vi "Database.GetProductComponentTable.vi"(5 "Idx":i32, 7 "ConnectionString":string, 8 "error in (no error)":errorcluster, 10 "Component_SerialNo":string, 11 "Component_WabcoNo":string) -> (0 "error out":errorcluster, 1 "Prod found":bool, 2 "Product_SerialNo":string, 3 "Product_WabcoNo":string)   [LabVIEW 2016]
uses:
  Tools/Translator/Translator.Message.ctl
  Tools/EventLog/EventLog.EventLevel.ctl
  Tools/EventLog/EventLog.EventSource.ctl
  Tools/EventLog/EventLog.New(array).vi
  <vilib>/addons/database/Connection.llb/DB Tools Open Connec (String).vi
  <vilib>/addons/database/Connection.llb/Conn Execute.vi
  <vilib>/addons/database/Recordset.llb/Rec Fetch Recordset Data (R).vi
  <vilib>/addons/database/Recordset.llb/Rec Destroy - Connection.vi
  Global/ApplicationGlobal.vi
  Tools/EventLog/EventLog.Buffer.vi
  Tools/EventLog/EventLog.File.ReadWrite.vi
  <vilib>/addons/database/NI_Database_API.lvlib
panel:
  in  "Data":i32(listbox)
  out "sql statement":string
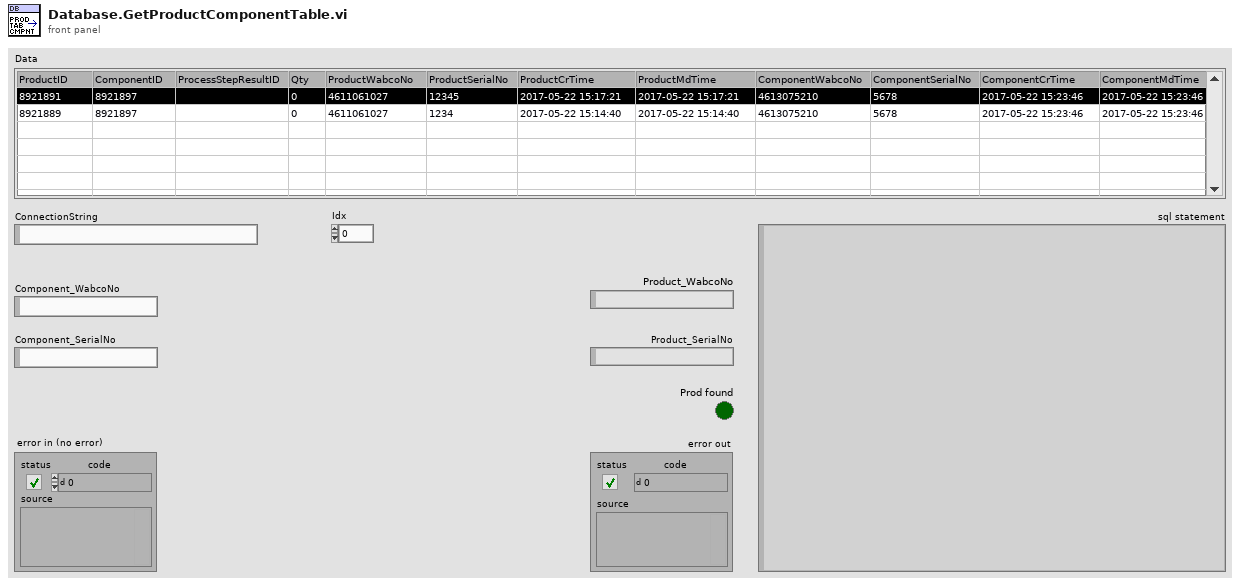
[diagram p1: front panel]
types:
  T1 = typedef "EventLog.EventSource.ctl" = enum16{"All", "Gui", "Cache", "PLC1", "PLC2", "PLC3", "DB", "DB01", "DB02", "DB03", "DB04", "DB05", "DB06", "DB07", "DB08", "DB09", "DB10", "DB11", "DB12", "DB13", "DB14", "DB15", "DB16"}
  T2 = typedef "EventLog.EventLevel.ctl" = enum8{"Debug", "Info", "Warning", "Error"}
  T3 = typedef "Translator.Message.ctl" = enum16{"-", "Event confirmed", "Log out", "Log in", "Shutdown", "Cancel", "Start", "Continue", "Stop", "On", "Off", "OK", "NOK", "NOK %s", "This", "Prev", "Home", "Work", "In progress...", "Missing", "Empty", "Hardware failure", "Initial", "Error %d >> %s", "Error %d >> %s >> %s", "Starting %s", "Quitting %s", "Configured", "Initializing", "Quitting", "Loading", "Running %s", "Stopped", "Summary", "Do you want to continue?", "Do you want to exit?", "Log out?", "System", "All", "IDLE", "Translating...%s", "Not found", "Alarm %s", "Run", "Skip", "Abort", "Repeat", "Please wait...", "Database disconnected", "Login to database successful", "Login to database failed: %d; %s", "Get process step data for %s", "Changeover off", "Changeover into %s", "Product %s | %s found in cache with status %d at previous station", "Product %s | %s found in database with status %d at previous station", "Product %s | %s not found in cache at previous station", "Product %s | %s not found in database at previous station", "Product %s | %s found in cache with status %d at this station (%d repetion)", "Product %s | %s found in database with status %d at this station (%d repetition)", "Product %s | %s not found in cache at this station", "Product %s | %s not found in database at this station", "Product %s | %s found in cache for component %s | %s", "Product %s | %s found in database for component %s | %s", "Product not found in cache for component %s | %s", "Product not found in database for component %s | %s", "Product %s | %s connected with component %s | %s (cache)", "Product %s | %s connected with component %s | %s (database)", "New data for %s | %s (cache)", "New data for %s | %s (database)", "File %s moved (cache)", "File %s deleted (cache)", "Msg %d >> %s", "PLC LifeBit Failure", "Reconnecting DB", "Reconnecting PLC", "Free disk space is below 1GB - contact technician"}
  T4 = typedef "NI_Database_API.lvlib/Conn ObjectReference.ctl" = refnum<k1>
  T5 = typedef "NI_Database_API.lvlib/Rec ObjectReference.ctl" = refnum<k1>
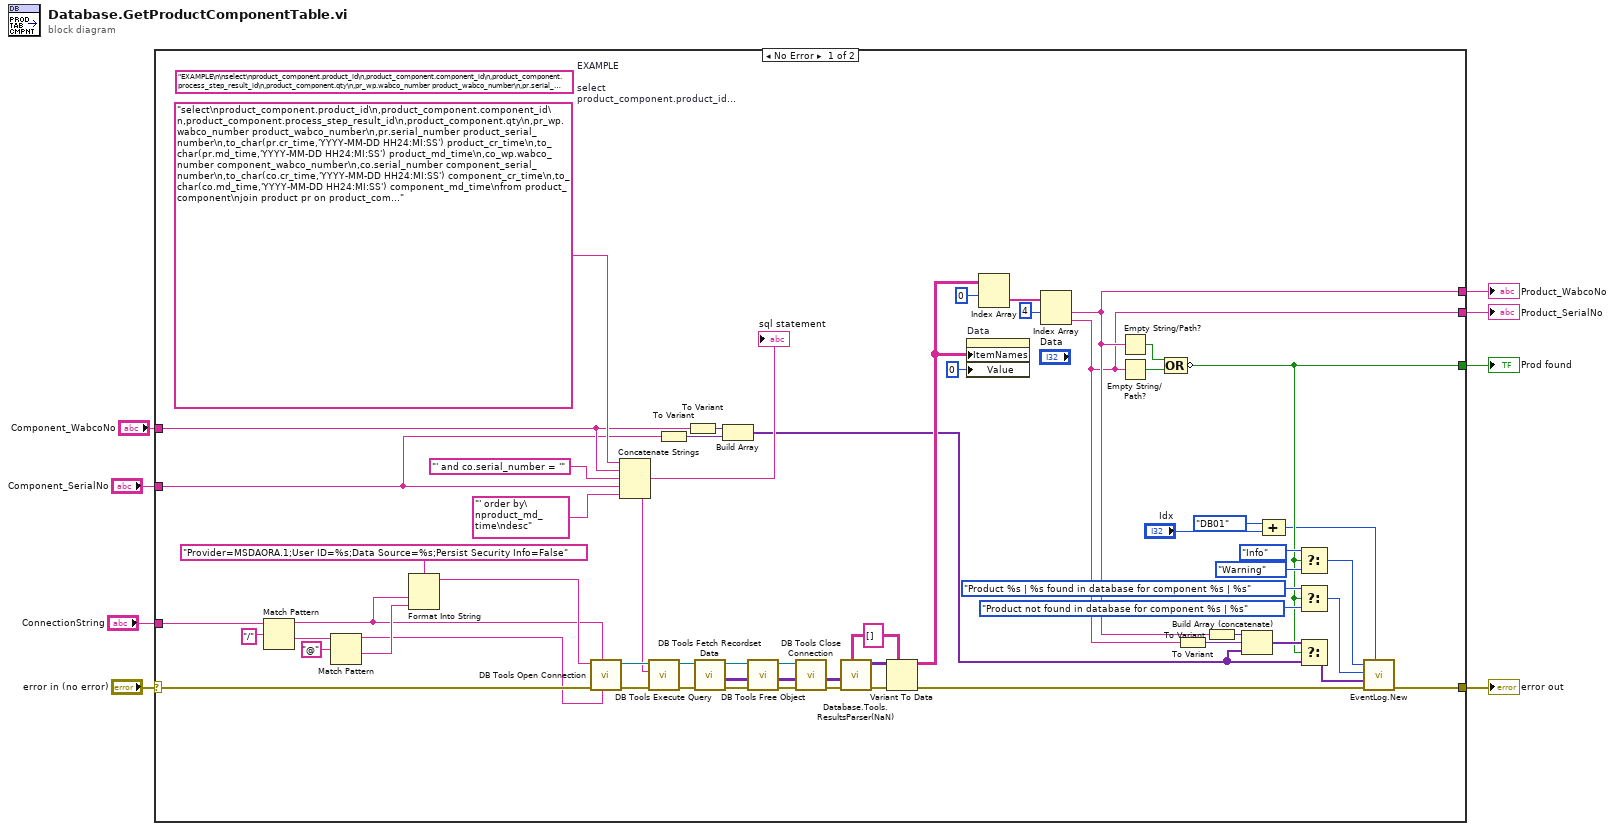
[diagram p0: block diagram]
diagram:
  n1 = case shown="No Error" "error in (no error)" {
    selector: "error in (no error)" -> [w54 w66]
    tunnel: "Component_SerialNo" -> [w14 _]
    tunnel: [w21 w66] -> w2
    tunnel: [w18 _] -> w7
    tunnel: [w19 _] -> w6
    tunnel: [w12 _] -> w5
    tunnel: "Component_WabcoNo" -> [w15 _]
    tunnel: "ConnectionString" -> [w49 _]
    frame No Error {
      w34 = string[][] [] ("Array")
      (unwired) "EXAMPLE\n\nselect\nproduct_component.product_id\n,product_component.component_id\n,product_component.process_step_result_id\n,product_component.qty\n,pr_wp.wabco_number product_wabco_number\n,pr.serial_number product_serial_number\n,to_char(pr.cr_time,'YYYY-MM-DD HH24:MI:SS') product_cr_time\n,to_char(pr.md_time,'YYYY-MM-DD HH24:MI:SS') product_md_time\n,co_wp.wabco_number component_wabco_number\n,co.serial_number component_serial_number\n,to_char(co.cr_time,'YYYY-MM-DD HH24:MI:SS') component_cr_time\n,to_char(co.md_time,'YYYY-MM-DD HH24:MI:SS') component_md_time\nfrom product_component\njoin product pr on product_component.product_id=pr.id\njoin wabcopart pr_wp on pr.wabco_part_id = pr_wp.id\njoin product co on product_component.component_id=co.id\njoin wabcopart co_wp on co.wabco_part_id = co_wp.id\nwhere \nco_wp.wabco_number = '4430203001'\nand co.serial_number = '03667'\norder by\nproduct_md_time\ndesc\n"  # EXAMPLE  select product_component.product_id ,product_component.component_id ,product_component.process_step_result_id ,product_component.qty ,pr_wp.wabco_number product_wabco_number ,pr.serial_number product_serial_number ,to_char(pr.cr_time,'YYYY-MM-DD HH24:MI:SS') product_cr_time ,to_char(pr.md_time,'YYYY-MM-DD HH24:MI:SS') product_md_time ,co_wp.wabco_number component_wabco_number ,co.serial_number component_serial_number ,to_char(co.cr_time,'YYYY-MM-DD HH24:MI:SS') component_cr_time ,to_char(co.md_time,'YYYY-MM-DD HH24:MI:SS') component_md_time from product_component join product pr on product_component.product_id=pr.id join wabcopart pr_wp on pr.wabco_part_id = pr_wp.id join product co on product_component.component_id=co.id join wabcopart co_wp on co.wabco_part_id = co_wp.id where  co_wp.wabco_number = '4430203001' and co.serial_number = '03667' order by product_md_time desc
      n2 = Match Pattern(string=w49, regular expression="/") -> (before substring=w45:string, after substring=w52:string)  [unwired: 1 in, 2 out]
      n3 = Match Pattern(string=w52, regular expression="@") -> (before substring=w44:string, after substring=w46:string)  [unwired: 1 in, 2 out]
      n4 = Format Into String(format string="Provider=MSDAORA.1;User ID=%s;Data Source=%s;Persist Security Info=False", w45, w46) -> (resulting string=w47:string)  [unwired: 2 in, 1 out]
      n5 = call-poly <vilib>:"DB Tools Open Connection.vi"("password"=w44, "userID"=w45, "error in (no error)"=w54, "connection information"=w47) -> ("error out"=w64:errorcluster, "connection reference"=w61:T4)  [unwired: 4 in]
      n6 = Concatenate Strings("select\nproduct_component.product_id\n,product_component.component_id\n,product_component.process_step_result_id\n,product_component.qty\n,pr_wp.wabco_number product_wabco_number\n,pr.serial_number product_serial_number\n,to_char(pr.cr_time,'YYYY-MM-DD HH24:MI:SS') product_cr_time\n,to_char(pr.md_time,'YYYY-MM-DD HH24:MI:SS') product_md_time\n,co_wp.wabco_number component_wabco_number\n,co.serial_number component_serial_number\n,to_char(co.cr_time,'YYYY-MM-DD HH24:MI:SS') component_cr_time\n,to_char(co.md_time,'YYYY-MM-DD HH24:MI:SS') component_md_time\nfrom product_component\njoin product pr on product_component.product_id=pr.id\njoin wabcopart pr_wp on pr.wabco_part_id = pr_wp.id\njoin product co on product_component.component_id=co.id\njoin wabcopart co_wp on co.wabco_part_id = co_wp.id\nwhere \nco_wp.wabco_number = '", w15, "' and co.serial_number = '", w14, "' order by\nproduct_md_time\ndesc") -> (w57:string)
      "sql statement" <- w57
      n7 = call-poly <vilib>:"DB Tools Execute Query.vi"("error in (no error)"=w64, "SQL query"=w57, "connection reference"=w61) -> ("error out"=w65:errorcluster, "recordset reference"=w62:T5)  [unwired: 5 in]
      n8 = To Variant(anything=w14) -> (Variant=w16:variant)
      n9 = To Variant(anything=w15) -> (Variant=w17:variant)
      n10 = call-poly <vilib>:"DB Tools Fetch Recordset Data.vi"("error in (no error)"=w65, "recordset reference"=w62) -> ("error out"=w38:errorcluster, "recordset data"=w33:variant[][], "recordset reference out"=w60:T5)  [unwired: 3 in]
      n11 = Build Array(w17, w16) -> (w13:variant[])
      n12 = call-poly <vilib>:"DB Tools Free Object.vi"("error in (no error)"=w38, "recordset reference"=w60) -> ("error out"=w63:errorcluster, "connection reference"=w59:T4)  [unwired: 8 in]
      n13 = call <vilib>:"DB Tools Close Connection.vi"("error in (no error)"=w63, "connection reference"=w59) -> ("error out"=w37:errorcluster)  [unwired: 5 in]
      n14 = call "Database.Tools.ResultsParser(NaN).vi"("Type"=w34, "error in (no error)"=w37, "Results in"=w33) -> ("error out"=w36:errorcluster, "Results out"=w35:variant[][])  [unwired: 7 in]
      n15 = Variant To Data(error in=w36, type=w34, Variant=w35) -> (data=w32:string[][], error out=w20:errorcluster)
      n16 = property on="Data" class="MCListbox (strict)"("ItemNames"=w32, "Value"=0 ("Data")) -> ()  [unwired: 2 in, 2 out]
      n17 = Index Array(array=w32, index (row)=0) -> (element=w42:string[])  [unwired: 1 in]
      n18 = Index Array(array=w42, index #1=4 ("disabled index (col)")) -> (element #1=w19:string, element #2=w18:string)  [unwired: 1 in]
      n19 = Empty String/Path?(string/path=w19) -> (empty?=w40:bool)
      n20 = Empty String/Path?(string/path=w18) -> (empty?=w53:bool)
      n21 = Compound Arithmetic op=OR(w40, w53) -> (invert w12:bool)
      n22 = To Variant(anything=w18) -> (Variant=w31:variant)
      n23 = To Variant(anything=w19) -> (Variant=w30:variant)
      n24 = Build Array (concatenate)(w30, w31, w13) -> (w29:variant[])
      n25 = Compound Arithmetic op=ADD(EventLog.EventSource."DB01" ("Source (All)"), "Idx") -> (w9:i32)
      n26 = Select(t=EventLog.EventLevel."Info" ("Level (Info)"), s=w12, f=EventLog.EventLevel."Warning" ("Level (Info)")) -> (s? t:f=w22:T2)
      n27 = Select(t=Translator.Message."Product %s | %s found in database for component %s | %s" ("Message (-)"), s=w12, f=Translator.Message."Product not found in database for component %s | %s" ("Message (-)")) -> (s? t:f=w26:T3)
      n28 = Select(t=w29, s=w12, f=w13) -> (s? t:f=w25:variant[])
      n29 = call-poly "EventLog.New.vi"("Source (All)"=w9, "error in (no error)"=w20, "Arguments"=w25, "Message (-)"=w26, "Level (Info)"=w22) -> ("error out"=w21:errorcluster)  [unwired: 5 in, 1 out]
    }
    frame Error {
    }
  }
  "Product_SerialNo" <- w7
  "Product_WabcoNo" <- w6
  "Prod found" <- w5
  "error out" <- w2
